vi "Get Channel Count Analog Out.vi"(8 "error in (no error)":errorcluster, 11 "hdwf":i32) -> (0 "error out":errorcluster, 2 "pcChannel":i32, 3 "hdwf out":i32)   [LabVIEW 2014, in "AnalogDiscSDKLv.lvlib"]
doc: "extern \"C\" __declspec(dllexport) int GetChannelCount_AnalogOut(\n HDWF hdwf,\n int *pcChannel\n );"
uses:
  <instrlib>/AnalogDiscSDKLv/AnalogDiscSDKLv.lvlib
  <instrlib>/AnalogDiscSDKLv/AnalogDiscSDKLv.dll
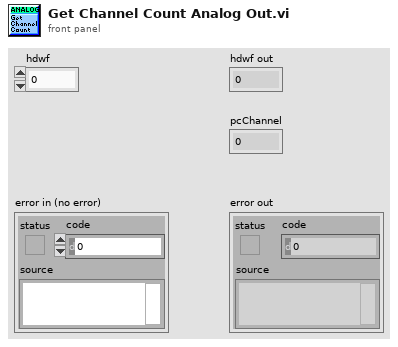
[diagram p1: front panel]
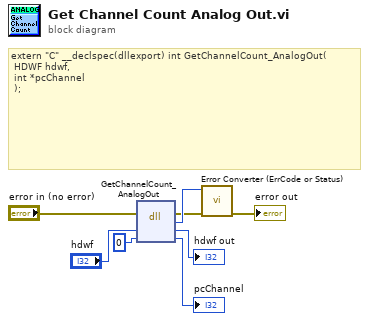
[diagram p0: block diagram]
diagram:
  # "extern \"C\" __declspec(dllexport) int GetChannelCount_AnalogOut(\n\tHDWF hdwf,\n\tint *pcChannel\n\t);"
  n1 = dll-call lib="C:/Program Files (x86)/National Instruments/LabVIEW 2014/instr.lib/AnalogDiscSDKLv/AnalogDiscSDKLv.*" fn="GetChannelCount_AnalogOut"(error in="error in (no error)", "hdwf"="hdwf", "pcChannel"=0) -> (error out=w2:errorcluster, w3:i32, "hdwf"=→"hdwf out":i32, "pcChannel"=→"pcChannel":i32)  [unwired: 2 in, 1 out]
  n2 = call <instrlib>:"Error Converter (ErrCode or Status).vi"("error in (no error)"=w2, "error code"=w3) -> ("error out"=→"error out":errorcluster)  [unwired: 9 in]
